vi "Ver 3.1.vi"() -> ()   [LabVIEW 2016]
doc: "This example VI shows how to use thermocouples to take a temperature measurement.\n\nNote:\nFor front panel measurements, make sure the Input switch is in the out position(F)\nFor plug-in card measurements, make sure the Input switch is in the in poisition(R)"
uses:
  Documents/keithley_27xx/Keithley 27XX/Keithley 27XX.lvlib
  Documents/keithley_27xx/Keithley 27XX/Public/Close.vi
  Documents/keithley_27xx/Keithley 27XX/Public/Data/Read Multiple Direct.vi
  Documents/keithley_27xx/Keithley 27XX/Public/Configure/Measurement Specific/Configure Thermocouple.vi
  Documents/keithley_27xx/Keithley 27XX/Public/Configure/Measurement Specific/Configure Thermistor.vi
  Documents/keithley_27xx/Keithley 27XX/Public/Configure/Measurement Specific/Configure FRTD.vi
panel:
  in  "Beta3":dbl=0.1
  in  "Alpha3":dbl=0.0038
  in  "Delta3":dbl=1.0
  in  "Beta2":dbl=0.1
  in  "Alpha2":dbl=0.0038
  in  "Delta2":dbl=1.0
  in  "Beta1":dbl=0.1
  in  "Alpha1":dbl=0.0038
  in  "Delta1":dbl=1.0
  out "Timestamp 12":dbl[](array[numeric])
  out "Timestamp 11":dbl[](array[numeric])
  out "Timestamp 10":dbl[](array[numeric])
  out "Timestamp 9":dbl[](array[numeric])
  out "Timestamp 8":dbl[](array[numeric])
  out "Timestamp 7":dbl[](array[numeric])
  out "Timestamp 6":dbl[](array[numeric])
  out "Timestamp 5":dbl[](array[numeric])
  out "Timestamp 4":dbl[](array[numeric])
  out "Timestamp 3":dbl[](array[numeric])
  out "Timestamp 2":dbl[](array[numeric])
  out "Measurement 12":dbl[](array[numeric])
  out "Measurement 11":dbl[](array[numeric])
  out "Measurement 10":dbl[](array[numeric])
  out "Measurement 9":dbl[](array[numeric])
  out "Measurement 8":dbl[](array[numeric])
  out "Measurement 7":dbl[](array[numeric])
  out "Measurement 6":dbl[](array[numeric])
  out "Measurement 5":dbl[](array[numeric])
  out "Measurement 4":dbl[](array[numeric])
  out "Measurement 3":dbl[](array[numeric])
  out "Measurement 2":dbl[](array[numeric])
  out "Timestamp 1":dbl[](array[numeric])
  out "Measurement 1":dbl[](array[numeric])
  in  "# of Channels":dbl=3.0
  in  "Sample size":dbl=3.0
  in  "Sensor Type":string(combo)="Thermistor"
  in  "Serial Configuration":T1={"Baud Rate (9600)"=9600, "Flow Control (1: XON/XOFF)"=1, "Termination Char (0:CR)"=0} {"Termination Char (0:CR)" items=["CR", "LF", "CRLF (Do not use)", "LFCR (Do not use)"]; "Flow Control (1: XON/XOFF)" items=["None", "XON/XOFF", "RTS/CTS (2701 Only)", "XON/XOFF & RTS/CTS (2701 Only)"]; "Baud Rate (9600)" items=["300"=300, "600"=600, "1200"=1200, "2400"=2400, "4800"=4800, "9600"=9600, "19.2k"=19200, "38.4k (2701 Only)"=38400, "57.6k (2701 Only)"=57600, "115.2k (2701 Only)"=115200]}
  in  "VISA resource name":refnum<visa-resource-name>="TCPIP0::192.168.69.200::1394::SOCKET"
  in  "Channels":string="101,102,103"
  in  "Temperature (0: Celsius)":u16(ring) items=["Celsius", "Fahrenheit", "Kelvin"]
  # "*For front panel measurements, make sure the Input switch is in the out position(F)*\n  For plug-in card measurements, make sure the Input switch is in the in position(R)"
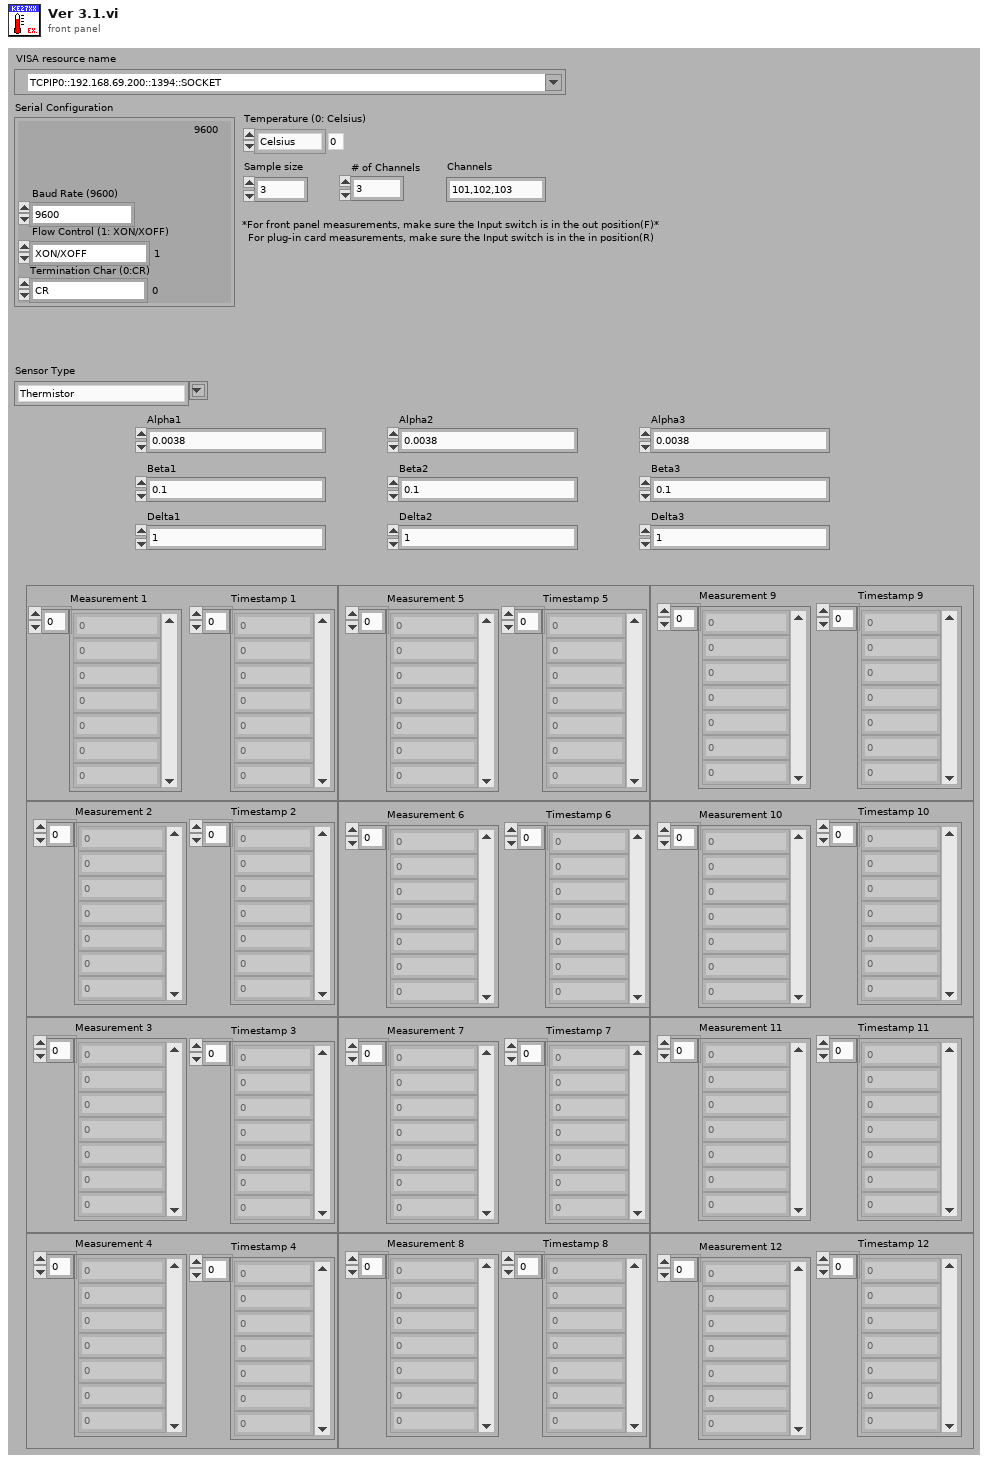
[diagram p1: front panel]
types:
  T1 = cluster{"Baud Rate (9600)":u32, "Flow Control (1: XON/XOFF)":u16, "Termination Char (0:CR)":u16}
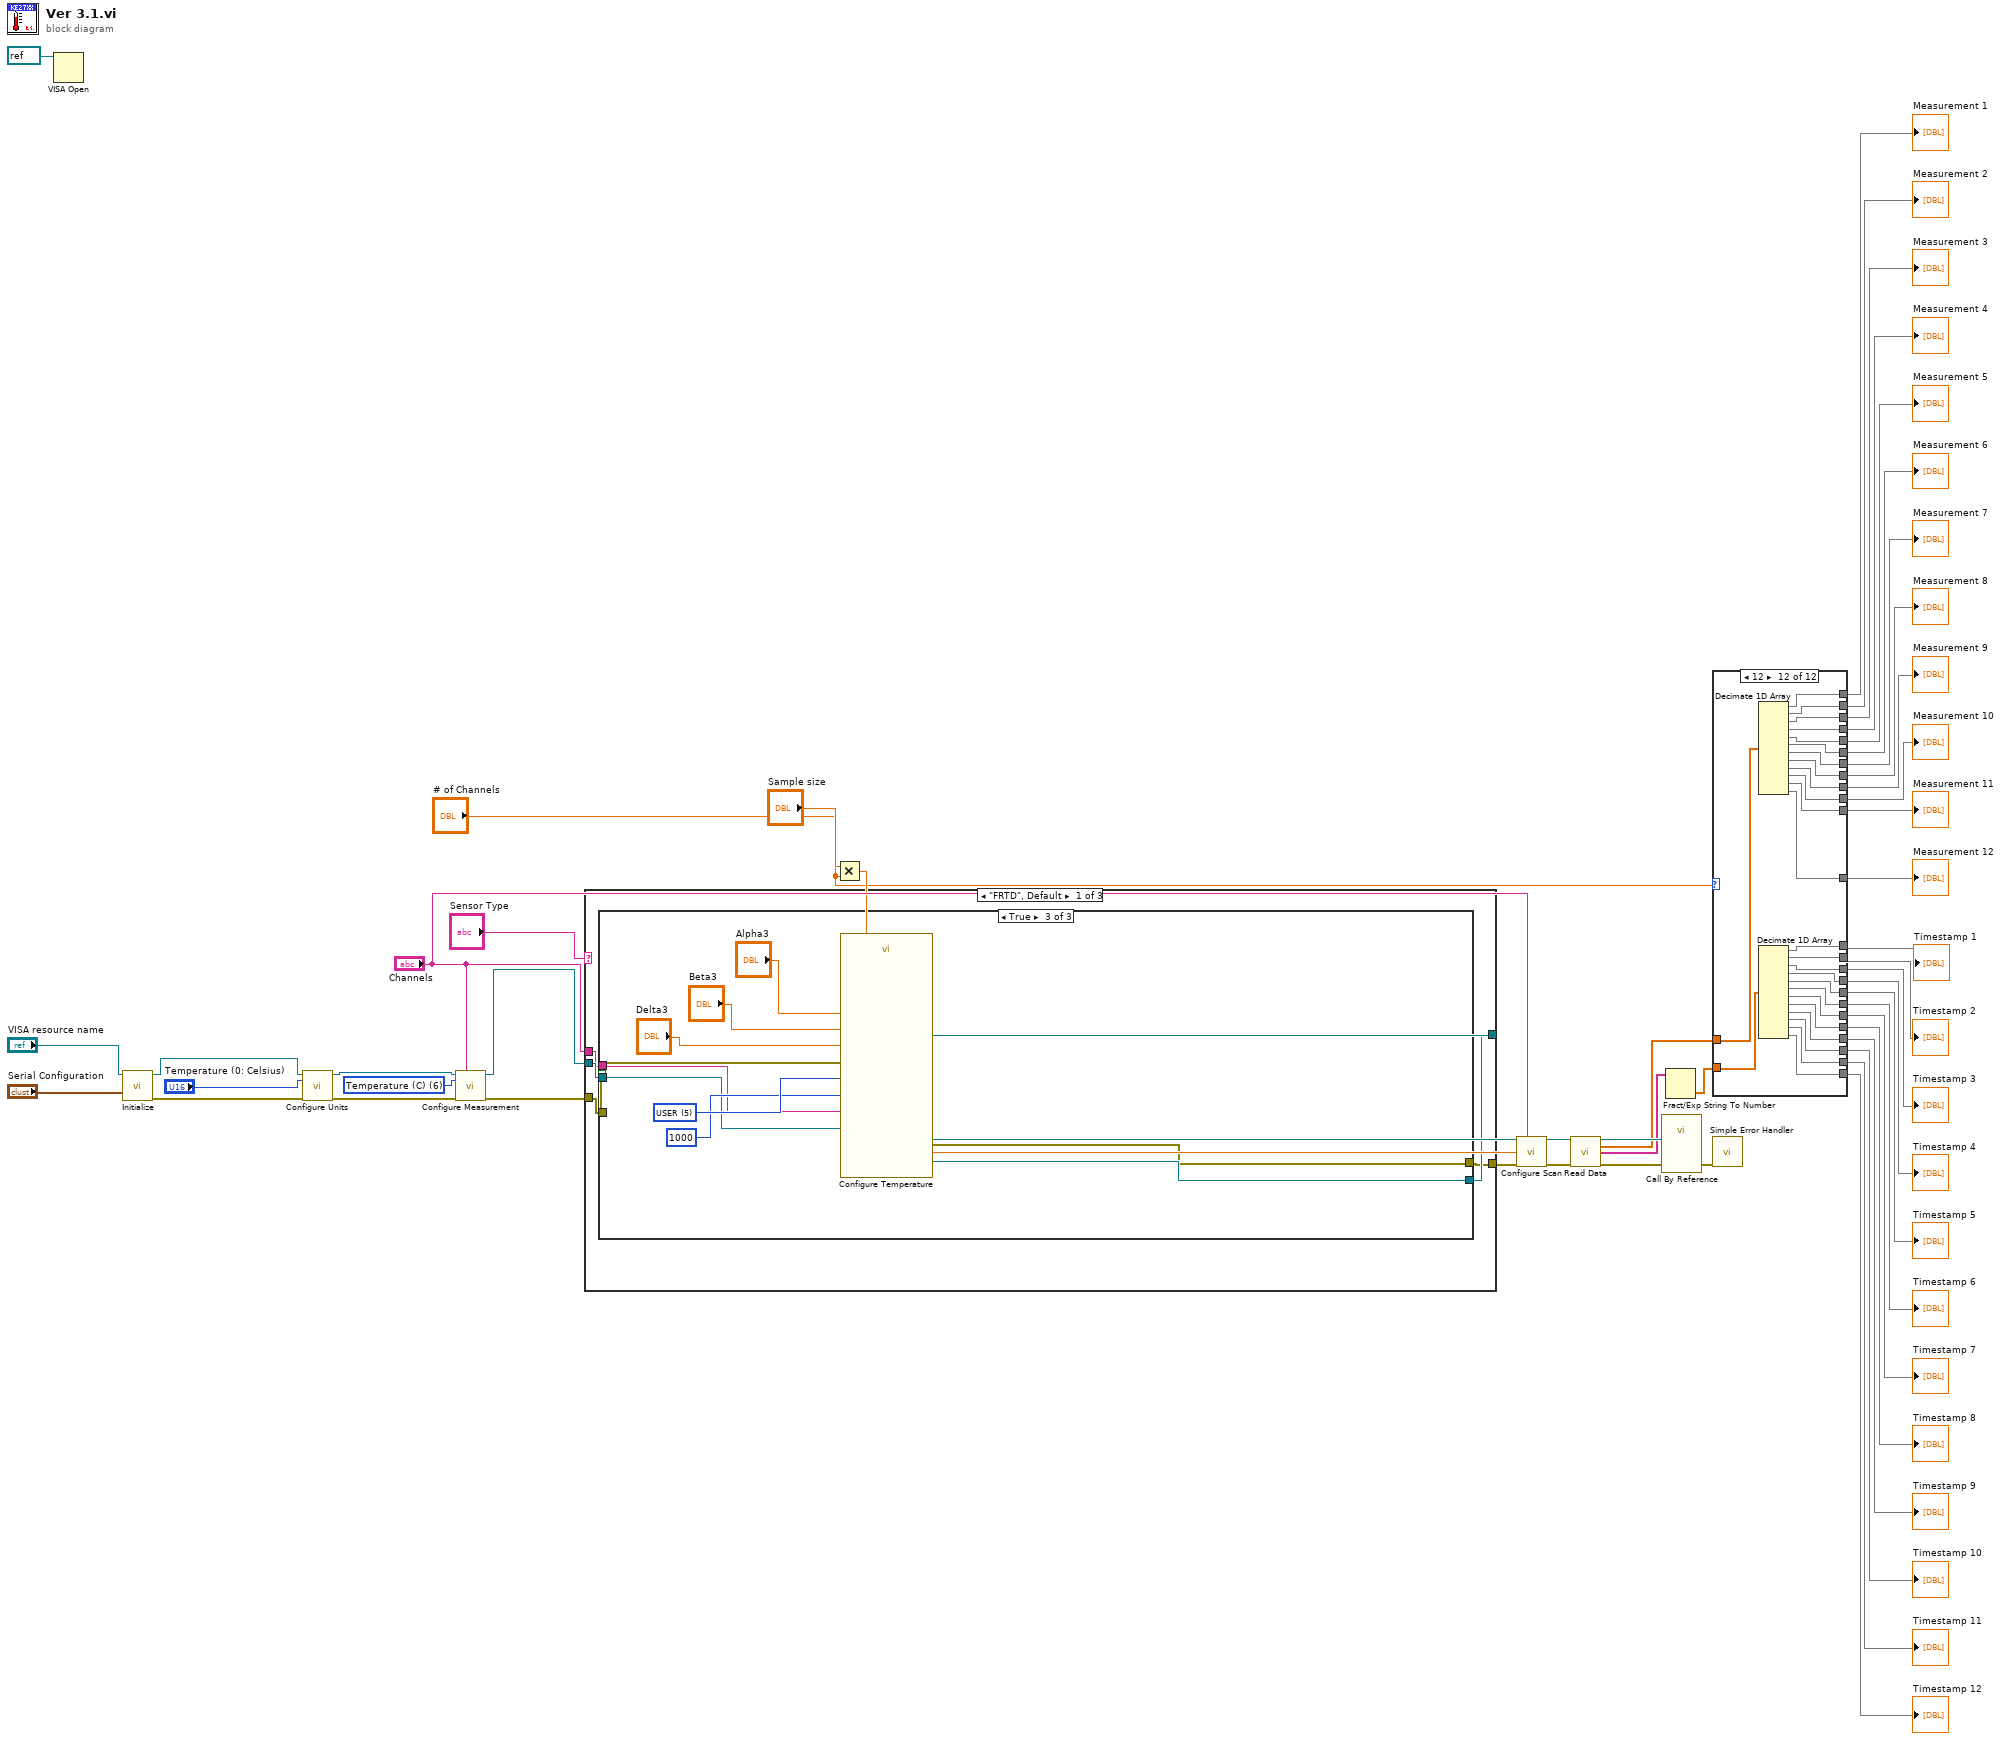
[diagram p0: block diagram]
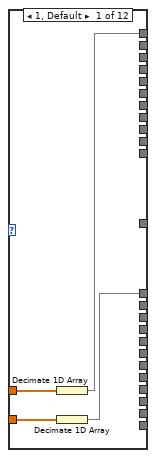
[diagram p2: hidden frame]
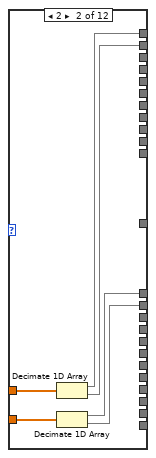
[diagram p3: hidden frame]
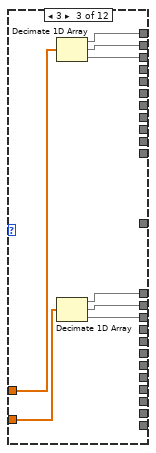
[diagram p4: hidden frame]
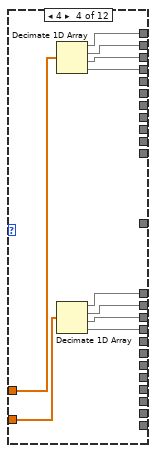
[diagram p5: hidden frame]
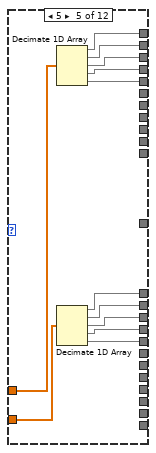
[diagram p6: hidden frame]
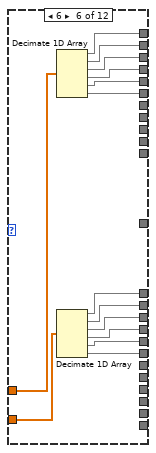
[diagram p7: hidden frame]
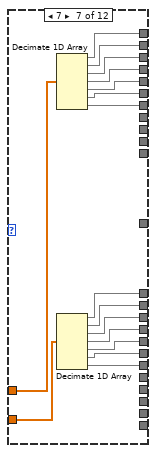
[diagram p8: hidden frame]
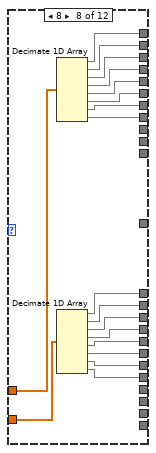
[diagram p9: hidden frame]
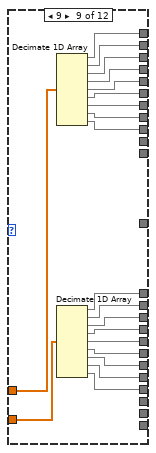
[diagram p10: hidden frame]
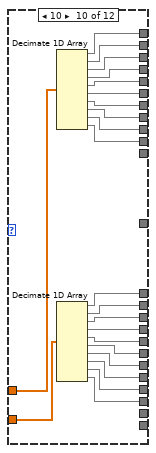
[diagram p11: hidden frame]
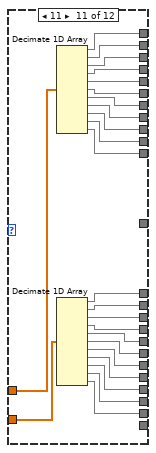
[diagram p12: hidden frame]
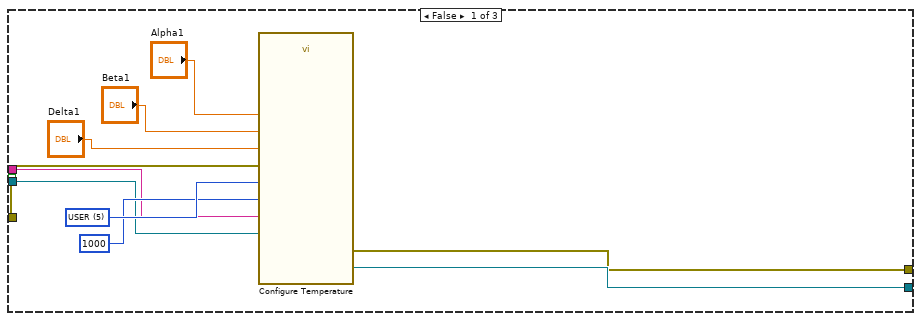
[diagram p13: hidden frame]
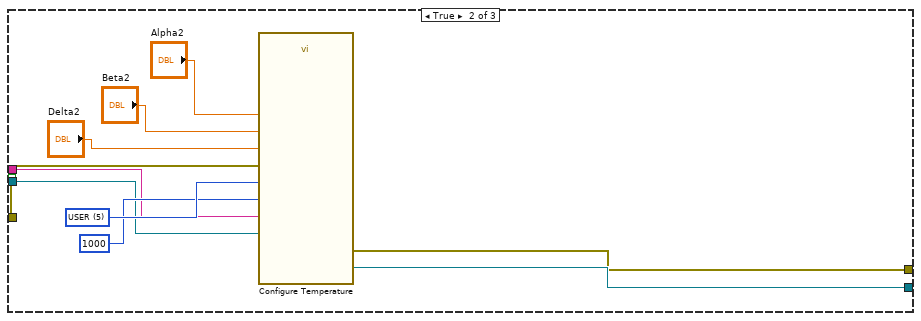
[diagram p14: hidden frame]
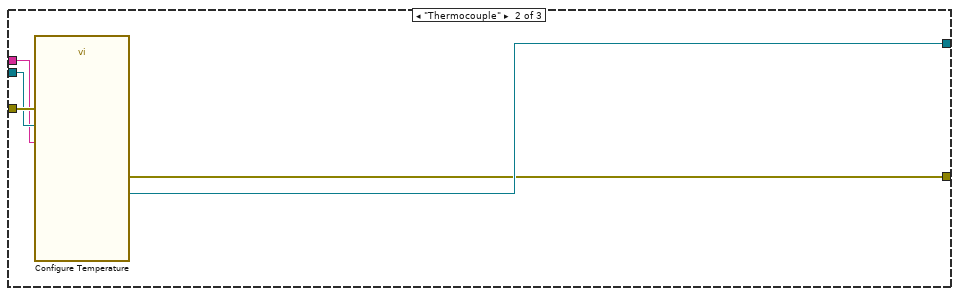
[diagram p15: hidden frame]
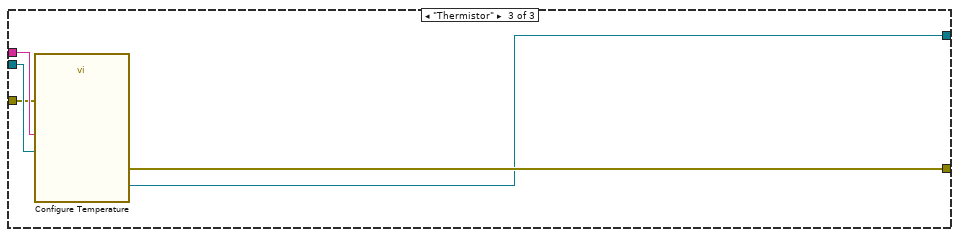
[diagram p16: hidden frame]
diagram:
  w48 = u16 6 items=["DC Voltage", "AC Voltage", "DC Current", "AC Current", "Resistance", "Four-Wire Resistance", "Temperature (C)", "Frequency", "Period", "Continuity"] ("Function (0: DC Voltage)")
  n1 = VISA Open(VISA resource name=refnum<visa-resource-name> refnum) -> ()  [unwired: 4 in, 2 out]
  n2 = call "Initialize.vi"("VISA resource name"="VISA resource name", "Serial Configuration"="Serial Configuration") -> ("VISA resource name out"=w45:refnum<visa-resource-name>, "error out"=w44:errorcluster)  [unwired: 12 in]
  n3 = call "Configure Units.vi"("VISA resource name"=w45, "Temperature (0: Celsius)"="Temperature (0: Celsius)", "error in (no error)"=w44) -> ("VISA resource name out"=w46:refnum<visa-resource-name>, "error out"=w43:errorcluster)  [unwired: 11 in]
  n4 = call "Configure Measurement.vi"("VISA resource name"=w46, "Scan List (Empty)"="Channels", "Function (0: DC Voltage)"=w48, "error in (no error)"=w43) -> ("VISA resource name out"=w38:refnum<visa-resource-name>, "error out"=w39:errorcluster)  [unwired: 10 in]
  n5 = case shown="\"FRTD\", Default" "Sensor Type" {
    tunnel: [w54 w89 w95] -> w41
    tunnel: [w55 w90 w94] -> w40
    tunnel: w39 -> [w53 w88 w91]
    tunnel: w38 -> [w52 w87 w92]
    tunnel: "Channels" -> [w51 w86 w93]
    frame "FRTD", Default {
      n6 = case shown="\"Channel 3\"" {
        selector: _ -> [_ _ _]
        tunnel: [w65 w75 w85] -> w55
        tunnel: [w64 w74 w84] -> w54
        tunnel: w53 -> [w61 w71 w81]
        tunnel: w52 -> [w60 w70 w80]
        tunnel: w51 -> [w59 w69 w79]
        frame False {
          w63 = u16 5 items=["PT100", "D100", "F100", "PT3916", "PT385", "USER"] ("FRTD Type (0: PT100)")
          n7 = call-poly "Configure Temperature.vi"("VISA resource name"=w60, "FRTD Type (0: PT100)"=w63, "error in (no error)"=w61, "Scan List (Empty)"=w59, "R Zero (100)"=1000, "Alpha (0.00385)"="Alpha1", "Beta (0.111)"="Beta1", "Delta (1.507)"="Delta1") -> ("VISA resource name out"=w65:refnum<visa-resource-name>, "error out"=w64:errorcluster)  [unwired: 10 in]
        }
        frame True {
          w73 = u16 5 items=["PT100", "D100", "F100", "PT3916", "PT385", "USER"] ("FRTD Type (0: PT100)")
          n8 = call-poly "Configure Temperature.vi"("VISA resource name"=w70, "FRTD Type (0: PT100)"=w73, "error in (no error)"=w71, "Scan List (Empty)"=w69, "R Zero (100)"=1000, "Alpha (0.00385)"="Alpha2", "Beta (0.111)"="Beta2", "Delta (1.507)"="Delta2") -> ("VISA resource name out"=w75:refnum<visa-resource-name>, "error out"=w74:errorcluster)  [unwired: 10 in]
        }
        frame True {
          w83 = u16 5 items=["PT100", "D100", "F100", "PT3916", "PT385", "USER"] ("FRTD Type (0: PT100)")
          n9 = call-poly "Configure Temperature.vi"("VISA resource name"=w80, "FRTD Type (0: PT100)"=w83, "error in (no error)"=w81, "Scan List (Empty)"=w79, "R Zero (100)"=1000, "Alpha (0.00385)"="Alpha3", "Beta (0.111)"="Beta3", "Delta (1.507)"="Delta3") -> ("VISA resource name out"=w85:refnum<visa-resource-name>, "error out"=w84:errorcluster)  [unwired: 10 in]
        }
      }
    }
    frame "Thermocouple" {
      n10 = call-poly "Configure Temperature.vi"("VISA resource name"=w87, "error in (no error)"=w88, "Scan List (Empty)"=w86) -> ("VISA resource name out"=w90:refnum<visa-resource-name>, "error out"=w89:errorcluster)  [unwired: 15 in]
    }
    frame "Thermistor" {
      n11 = call-poly "Configure Temperature.vi"("VISA resource name"=w92, "error in (no error)"=w91, "Scan List (Empty)"=w93) -> ("VISA resource name out"=w94:refnum<visa-resource-name>, "error out"=w95:errorcluster)  [unwired: 15 in]
    }
  }
  n12 = Multiply(x="Sample size", y="# of Channels") -> (x*y=w29:dbl)
  n13 = call "Configure Scan.vi"("VISA resource name"=w40, "Channel List (101:110)"="Channels", "Sample Count (100)"=w29, "error in (no error)"=w41) -> ("VISA resource name out"=w34:refnum<visa-resource-name>, "error out"=w33:errorcluster)  [unwired: 10 in]
  n14 = call-poly "Read Data.vi"("VISA resource name"=w34, "error in (no error)"=w33) -> ("VISA resource name out"=w32:refnum<visa-resource-name>, "Measurement Data"=w31:dbl[], "Time Stamp"=w15:string[], "error out"=w28:errorcluster)  [unwired: 8 in, 2 out]
  n15 = call-by-ref "?"("VISA resource name"=w32, "error in (no error)"=w28) -> ("error out"=w35:errorcluster)  [unwired: 15 in, 2 out]
  n16 = Fract/Exp String To Number(string=w15) -> (number=w26:dbl[])  [unwired: 3 in, 1 out]
  n17 = case shown="12" "# of Channels" {
    tunnel: w26 -> [w99 w104 w112 w122 w134 w148 w164 w182 w202 w224 w248 w274]
    tunnel: w31 -> [w98 w105 w113 w123 w135 w149 w165 w183 w203 w225 w249 w275]
    tunnel: [w97 w103 w111 w121 w133 w147 w163 w181 w201 w223 w247 w273] -> w25
    tunnel: [w96 w102 w108 w118 w130 w144 w160 w178 w198 w220 w244 w270] -> w24
    tunnel: [_ w101 w110 w120 w132 w146 w162 w180 w200 w222 w246 w272] -> w23
    tunnel: [_ w100 w107 w117 w129 w143 w159 w177 w197 w219 w243 w269] -> w22
    tunnel: [_ _ w109 w119 w131 w145 w161 w179 w199 w221 w245 w271] -> w21
    tunnel: [_ _ w106 w116 w128 w142 w158 w176 w196 w218 w242 w268] -> w20
    tunnel: [_ _ _ w115 w127 w141 w157 w175 w195 w217 w241 w267] -> w19
    tunnel: [_ _ _ w114 w126 w140 w156 w174 w194 w216 w240 w266] -> w18
    tunnel: [_ _ _ _ w125 w139 w155 w173 w193 w215 w239 w265] -> w17
    tunnel: [_ _ _ _ w124 w138 w154 w172 w192 w214 w238 w264] -> w16
    tunnel: [_ _ _ _ _ w137 w153 w171 w191 w213 w237 w263] -> w14
    tunnel: [_ _ _ _ _ w136 w152 w170 w190 w212 w236 w262] -> w13
    tunnel: [_ _ _ _ _ _ w151 w169 w189 w211 w235 w261] -> w12
    tunnel: [_ _ _ _ _ _ w150 w168 w188 w210 w234 w260] -> w11
    tunnel: [_ _ _ _ _ _ _ w167 w187 w209 w233 w259] -> w10
    tunnel: [_ _ _ _ _ _ _ w166 w186 w208 w232 w258] -> w9
    tunnel: [_ _ _ _ _ _ _ _ w185 w207 w231 w257] -> w8
    tunnel: [_ _ _ _ _ _ _ _ w184 w206 w230 w256] -> w7
    tunnel: [_ _ _ _ _ _ _ _ _ w205 w229 w255] -> w6
    tunnel: [_ _ _ _ _ _ _ _ _ w204 w228 w254] -> w5
    tunnel: [_ _ _ _ _ _ _ _ _ _ w227 w253] -> w4
    tunnel: [_ _ _ _ _ _ _ _ _ _ w226 w252] -> w3
    tunnel: [_ _ _ _ _ _ _ _ _ _ _ w251] -> w2
    tunnel: [_ _ _ _ _ _ _ _ _ _ _ w250] -> w1
    frame 1, Default {
      n18 = Decimate 1D Array(w98) -> (w97:dbl[])
      n19 = Decimate 1D Array(w99) -> (w96:dbl[])
    }
    frame 2 {
      n20 = Decimate 1D Array(w105) -> (w103:dbl[], w101:dbl[])
      n21 = Decimate 1D Array(w104) -> (w102:dbl[], w100:dbl[])
    }
    frame 3 {
      n22 = Decimate 1D Array(w113) -> (w111:dbl[], w110:dbl[], w109:dbl[])
      n23 = Decimate 1D Array(w112) -> (w108:dbl[], w107:dbl[], w106:dbl[])
    }
    frame 4 {
      n24 = Decimate 1D Array(w123) -> (w121:dbl[], w120:dbl[], w119:dbl[], w115:dbl[])
      n25 = Decimate 1D Array(w122) -> (w118:dbl[], w117:dbl[], w116:dbl[], w114:dbl[])
    }
    frame 5 {
      n26 = Decimate 1D Array(w135) -> (w133:dbl[], w132:dbl[], w131:dbl[], w127:dbl[], w125:dbl[])
      n27 = Decimate 1D Array(w134) -> (w130:dbl[], w129:dbl[], w128:dbl[], w126:dbl[], w124:dbl[])
    }
    frame 6 {
      n28 = Decimate 1D Array(w149) -> (w147:dbl[], w146:dbl[], w145:dbl[], w141:dbl[], w139:dbl[], w137:dbl[])
      n29 = Decimate 1D Array(w148) -> (w144:dbl[], w143:dbl[], w142:dbl[], w140:dbl[], w138:dbl[], w136:dbl[])
    }
    frame 7 {
      n30 = Decimate 1D Array(w165) -> (w163:dbl[], w162:dbl[], w161:dbl[], w157:dbl[], w155:dbl[], w153:dbl[], w151:dbl[])
      n31 = Decimate 1D Array(w164) -> (w160:dbl[], w159:dbl[], w158:dbl[], w156:dbl[], w154:dbl[], w152:dbl[], w150:dbl[])
    }
    frame 8 {
      n32 = Decimate 1D Array(w183) -> (w181:dbl[], w180:dbl[], w179:dbl[], w175:dbl[], w173:dbl[], w171:dbl[], w169:dbl[], w167:dbl[])
      n33 = Decimate 1D Array(w182) -> (w178:dbl[], w177:dbl[], w176:dbl[], w174:dbl[], w172:dbl[], w170:dbl[], w168:dbl[], w166:dbl[])
    }
    frame 9 {
      n34 = Decimate 1D Array(w203) -> (w201:dbl[], w200:dbl[], w199:dbl[], w195:dbl[], w193:dbl[], w191:dbl[], w189:dbl[], w187:dbl[], w185:dbl[])
      n35 = Decimate 1D Array(w202) -> (w198:dbl[], w197:dbl[], w196:dbl[], w194:dbl[], w192:dbl[], w190:dbl[], w188:dbl[], w186:dbl[], w184:dbl[])
    }
    frame 10 {
      n36 = Decimate 1D Array(w225) -> (w223:dbl[], w222:dbl[], w221:dbl[], w217:dbl[], w215:dbl[], w213:dbl[], w211:dbl[], w209:dbl[], w207:dbl[], w205:dbl[])
      n37 = Decimate 1D Array(w224) -> (w220:dbl[], w219:dbl[], w218:dbl[], w216:dbl[], w214:dbl[], w212:dbl[], w210:dbl[], w208:dbl[], w206:dbl[], w204:dbl[])
    }
    frame 11 {
      n38 = Decimate 1D Array(w249) -> (w247:dbl[], w246:dbl[], w245:dbl[], w241:dbl[], w239:dbl[], w237:dbl[], w235:dbl[], w233:dbl[], w231:dbl[], w229:dbl[], w227:dbl[])
      n39 = Decimate 1D Array(w248) -> (w244:dbl[], w243:dbl[], w242:dbl[], w240:dbl[], w238:dbl[], w236:dbl[], w234:dbl[], w232:dbl[], w230:dbl[], w228:dbl[], w226:dbl[])
    }
    frame 12 {
      n40 = Decimate 1D Array(w275) -> (w273:dbl[], w272:dbl[], w271:dbl[], w267:dbl[], w265:dbl[], w263:dbl[], w261:dbl[], w259:dbl[], w257:dbl[], w255:dbl[], w253:dbl[], w251:dbl[])
      n41 = Decimate 1D Array(w274) -> (w270:dbl[], w269:dbl[], w268:dbl[], w266:dbl[], w264:dbl[], w262:dbl[], w260:dbl[], w258:dbl[], w256:dbl[], w254:dbl[], w252:dbl[], w250:dbl[])
    }
  }
  "Measurement 1" <- w25
  "Timestamp 1" <- w24
  "Measurement 2" <- w23
  "Measurement 3" <- w21
  "Measurement 4" <- w19
  "Measurement 5" <- w17
  "Measurement 6" <- w14
  "Measurement 7" <- w12
  "Measurement 8" <- w10
  "Measurement 9" <- w8
  "Measurement 10" <- w6
  "Measurement 11" <- w4
  "Measurement 12" <- w2
  "Timestamp 2" <- w22
  "Timestamp 3" <- w20
  "Timestamp 4" <- w18
  "Timestamp 5" <- w16
  "Timestamp 6" <- w13
  "Timestamp 7" <- w11
  "Timestamp 8" <- w9
  "Timestamp 9" <- w7
  "Timestamp 10" <- w5
  "Timestamp 11" <- w3
  "Timestamp 12" <- w1
  n42 = call <vilib>:"Simple Error Handler.vi"("error in (no error)"=w35) -> ()  [unwired: 4 in, 5 out]
